vi "Add Keyboard.vi"(7 "Note Length (-1)":dbl=-1.0, 8 "error in (no error)":errorcluster, 10 "Position":enum16{"Top", "Left", "Botom", "Right"}(ring), 11 "midi-ui in":refnum<class "midi-ui.lvclass">) -> (0 "error out":errorcluster, 3 "midi-ui out":refnum<class "midi-ui.lvclass">)   [LabVIEW 2020, in "midi-ui.lvclass"]
uses:
  midi-ui.lvclass
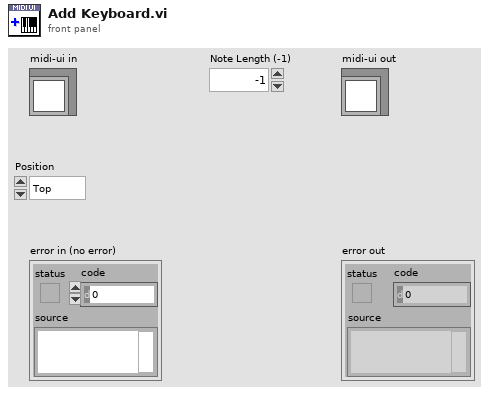
[diagram p1: front panel]
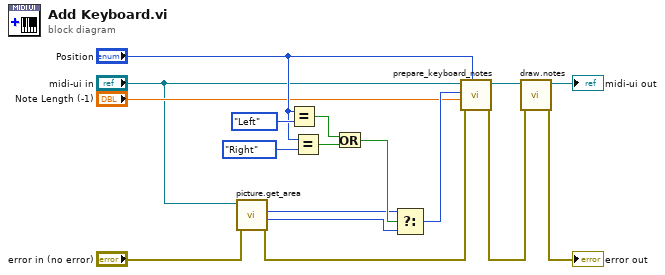
[diagram p0: block diagram]
diagram:
  n1 = call "picture.get_area.vi"("error in (no error)"="error in (no error)", "midi-ui in"="midi-ui in") -> ("error out"=w1:errorcluster, "Bounds:Area Width"=w4:u32, "Bounds:Area Height"=w5:u32)  [unwired: 6 in, 1 out]
  n2 = Equal?(x="Position", y=enum16{"Top", "Left", "Botom", "Right"}."Left") -> (x = y?=w15:bool)
  n3 = Equal?(x="Position", y=enum16{"Top", "Left", "Botom", "Right"}."Right") -> (x = y?=w14:bool)
  n4 = Or(x=w15, y=w14) -> (x .or. y?=w12:bool)
  n5 = Select(t=w5, s=w12, f=w4) -> (s? t:f=w11:u32)
  n6 = call "prepare_keyboard_notes.vi"("Anticlockwise rotations [0-3] (0)"="Position", "error in (no error)"=w1, "Note Length (-1)"="Note Length (-1)", "Total Length (1200)"=w11, "midi-ui in"="midi-ui in") -> ("error out"=w8:errorcluster, "midi-ui out"=w10:refnum<class "midi-ui.lvclass">)  [unwired: 5 in]
  n7 = call "draw.notes.vi"("error in (no error)"=w8, "midi-ui in"=w10) -> ("error out"=→"error out":errorcluster, "midi-ui out"=→"midi-ui out":refnum<class "midi-ui.lvclass">)  [unwired: 8 in]
